vi "AMZ_S3_APIHLP_Parse Delete Object Result for VersioningData.vi"(8 "error in (no error)":errorcluster, 11 "Response header":string) -> (0 "error out":errorcluster, 3 "Versioning Data":T1)   [LabVIEW 2015, in "LV Interface for Amazon S3.lvlib"]
uses:
  LV Interface for Amazon S3.lvlib
  Typedefs/AMZ_S3_API_Delete Object with Versioning Result.ctl
  <vilib>/regexp/Match Regular Expression.xnode
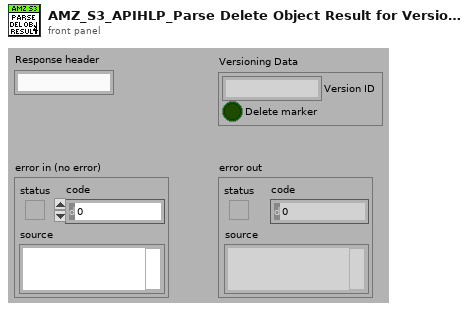
[diagram p1: front panel]
types:
  T1 = typedef "LV Interface for Amazon S3.lvlib/AMZ_S3_API_Delete Object with Versioning Result.ctl" = cluster{"Version ID":string, "Delete marker":bool}
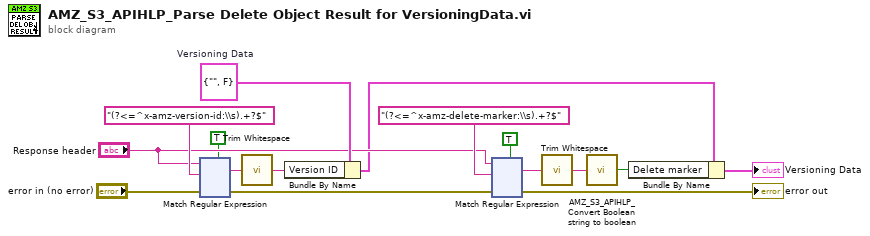
[diagram p0: block diagram]
diagram:
  w14 = T1 {"Version ID"="", "Delete marker"=FALSE}  # Versioning Data
  n1 = xnode "Match Regular Expression"("input string"="Response header", "regular expression"="(?<=^x-amz-version-id:\\s).+?$", "error in"="error in (no error)", "multiline? (F)"=TRUE) -> ("whole match"=w4:string, "error out"=w12:errorcluster)  [unwired: 2 in, 3 out]
  n2 = call <vilib>:"Trim Whitespace.vi"("string"=w4) -> ("trimmed string"=w3:string)  [unwired: 1 in]
  n3 = Bundle By Name(cluster=w14, "Version ID"=w3) -> (w10:T1)
  n4 = xnode "Match Regular Expression"("input string"="Response header", "regular expression"="(?<=^x-amz-delete-marker:\\s).+?$", "error in"=w12, "multiline? (F)"=TRUE) -> ("whole match"=w1:string, "error out"=→"error out":errorcluster)  [unwired: 2 in, 3 out]
  n5 = call <vilib>:"Trim Whitespace.vi"("string"=w1) -> ("trimmed string"=w2:string)  [unwired: 1 in]
  n6 = call "AMZ_S3_APIHLP_Convert Boolean string to boolean.vi"("Boolean string in"=w2) -> ("Boolean out"=w9:bool)  [unwired: 4 in]
  n7 = Bundle By Name(cluster=w10, "Delete marker"=w9) -> (→"Versioning Data":T1)
